vi "report.vi"(9 "Luxshare_P/N:":string="L12345678", 10 "SystemMode":string="GPF001", 11 "TXT path":string) -> ()   [LabVIEW 2011]
panel:
  out "Report Name":string
  out "x-y":u32
  out "Project  Information":string[][](array[string])
  in  "Report Type:":u16(ring) items=["Excel", "Excel&PDF"]
  in  "End Page":i32=3
  in  "Start Page":i32=1
  out "数组":string[](array[string])
  out "Report Config":string[](array[string])
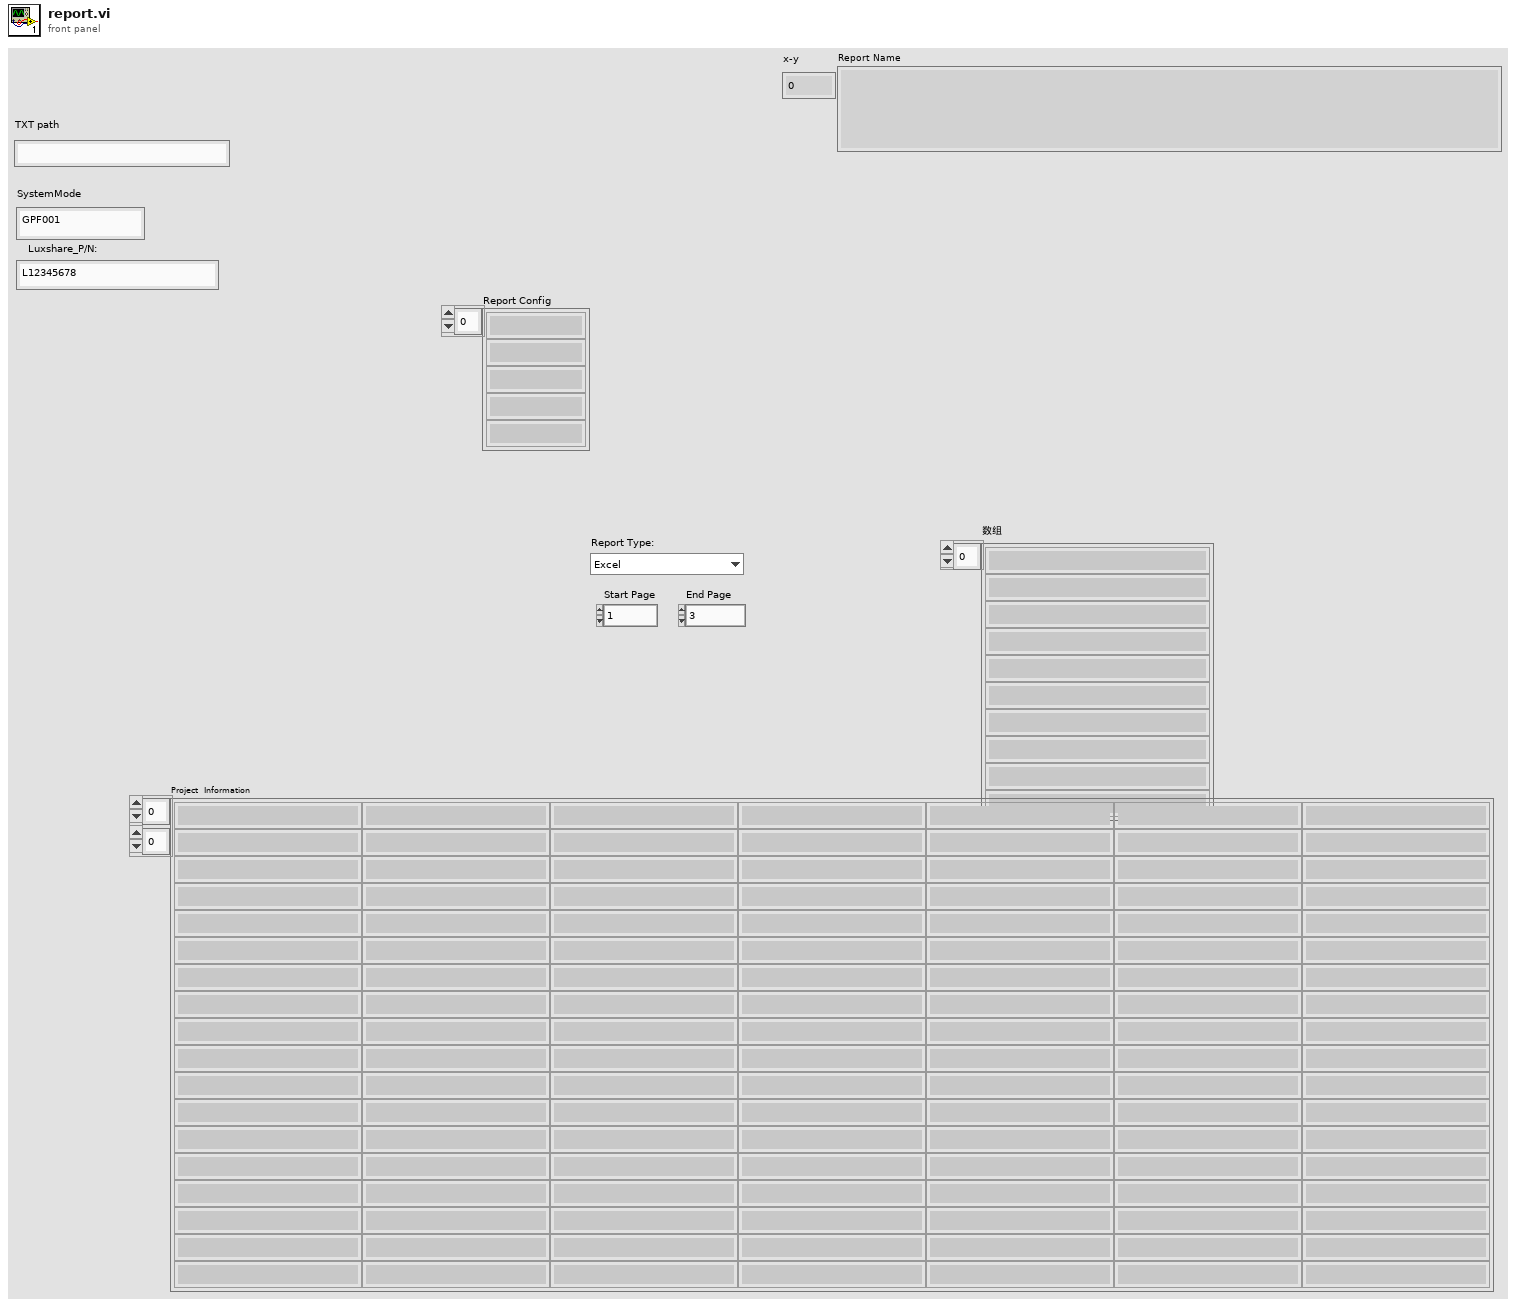
[diagram p1: front panel]
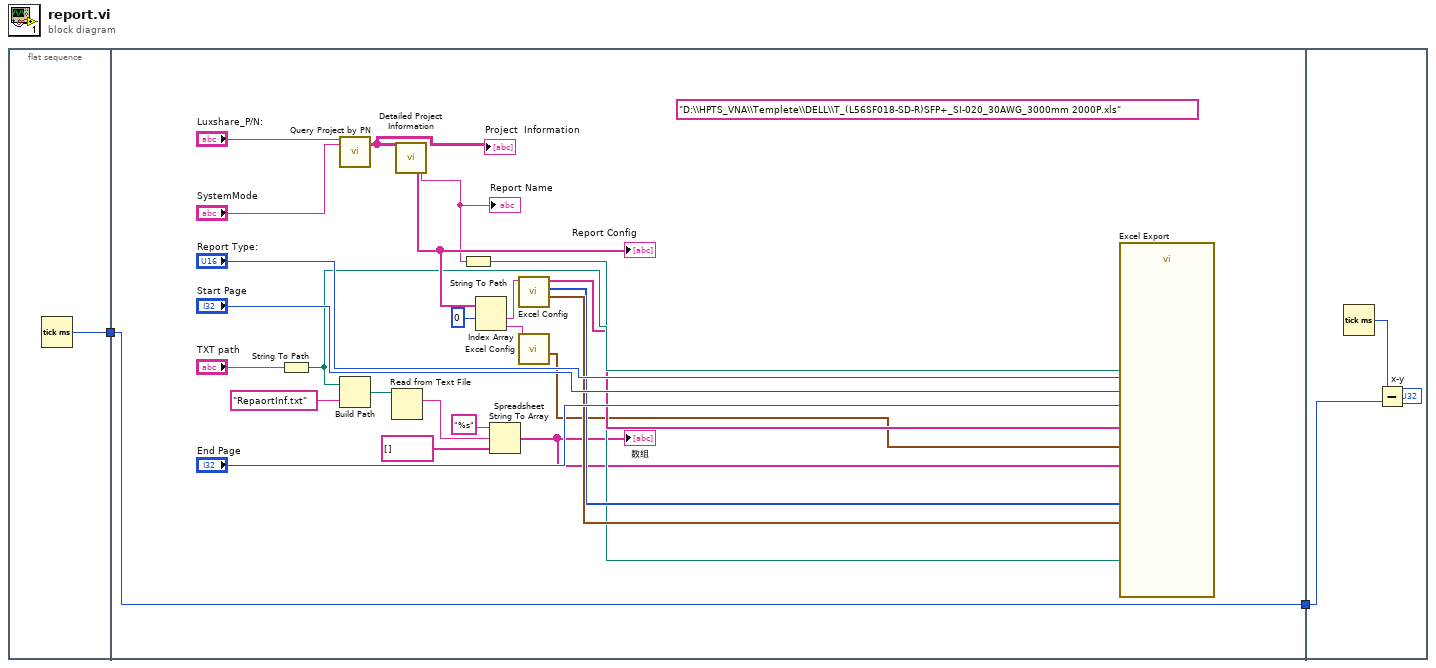
[diagram p0: block diagram]
diagram:
  n1 = flat-sequence {
    tunnel: [w3] -> w2
    tunnel: w2 -> [w5]
    tunnel: [w5] -> w1
    tunnel: w1 -> [w30]
    frame #0 {
      n2 = Tick Count (ms)() -> (millisecond timer value=w3:u32)
    }
    frame #1 {
      (unwired) "D:\\HPTS_VNA\\Templete\\DELL\\T_(L56SF018-SD-R)SFP+_SI-020_30AWG_3000mm 2000P.xls" ("Report Name")
      n3 = String To Path(string="TXT path") -> (path=w20:path)
      n4 = call "Query Project by PN.vi"("Luxshare_P/N:"="Luxshare_P/N:", "System_Mode"="SystemMode") -> ("Project  Information"=w26:string[][])  [unwired: 11 in, 6 out]
      "Project  Information" <- w26
      n5 = Build Path(base path=w20, name or relative path="RepaortInf.txt" ("名称或相对路径")) -> (appended path=w9:path)
      n6 = Read from Text File(file (use dialog)=w9) -> (text=w8:string)  [unwired: 3 in, 3 out]
      n7 = call "Detailed Project Information.vi"("Project  Information Input"=w26) -> ("Report Config"=w25:string[], "Report Name"=w4:string)  [unwired: 11 in, 14 out]
      "Report Config" <- w25
      "Report Name" <- w4
      n8 = String To Path(string=w4) -> (path=w16:path)
      n9 = Index Array(array=w25, index #1=0 ("索引")) -> (element #1=w14:string, element #2=w13:string)  [unwired: 1 in]
      n10 = Spreadsheet String To Array(format string="%s" ("格式字符串"), spreadsheet string=w8, array type (2D Dbl)=string[] [] ("添加的数组")) -> (array=w11:string[])  [unwired: 1 in]
      "数组" <- w11
      n11 = call "Excel Config.vi"("Config String"=w14) -> ("Start(0,0)"=w19:cluster{i32, i32}[], "Sheet Number List"=w18:i32[], "File Name List"=w17:string[])  [unwired: 8 in]
      n12 = call "Excel Config.vi"("Config String"=w13) -> ("Start(0,0)"=w12:cluster{i32, i32}[])  [unwired: 8 in, 2 out]
      n13 = call "Excel Export.vi"("template Path"=w16, "Data Basic Path"=w20, "File Name List"=w17, "Sheet Index List"=w18, "Report Inf"=w11, "Inf start"=w12, "Sheet start(0,0)"=w19, "Report Type"="Report Type:", "StartPage"="Start Page", "EndPage"="End Page") -> ()  [unwired: 17 in, 1 out]
    }
    frame #2 {
      n14 = Tick Count (ms)() -> (millisecond timer value=w31:u32)
      n15 = Subtract(x=w31, y=w30) -> (x-y=→"x-y":u32)
    }
  }
